vi "AddCustomError.vi"(1 "error in (no error)":errorcluster, 2 "source":string, 3 "code":i32, 4 "Error?":bool) -> (0 "error in (no error) 2":errorcluster)   [LabVIEW 2013]
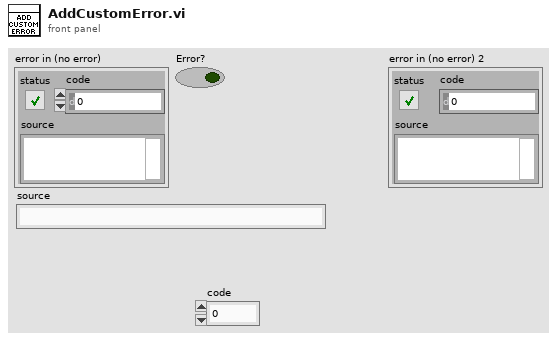
[diagram p1: front panel]
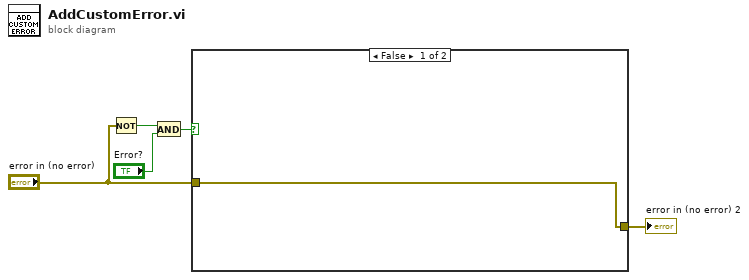
[diagram p0: block diagram]
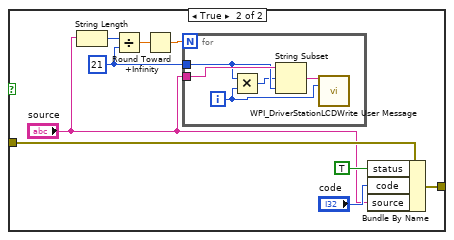
[diagram p2: hidden frame]
diagram:
  n1 = Not(x="error in (no error)") -> (.not. x?=w4:bool)
  n2 = And(x=w4, y="Error?") -> (x .and. y?=w5:bool)
  n3 = case shown="False" w5 {
    tunnel: "error in (no error)" -> [w6 w15]
    tunnel: [w6 w13] -> w1
    frame False {
    }
    frame True {
      w7 = 21 ("y")
      n4 = String Length(string="source") -> (length=w11:i32)
      n5 = Divide(x=w11, y=w7) -> (x/y=w10:dbl)
      n6 = Round Toward +Infinity(x=w10) -> (ceil(x): smallest int >= x=w9:dbl)
      n7 = for {
        N: w9 -> [_]
        tunnel: "source" -> [w20]
        tunnel: w7 -> [w19]
        i -> [w18]
        n8 = Multiply(x=w19, y=w18) -> (x*y=w17:i32)
        n9 = String Subset(string=w20, offset (0)=w17, length (rest)=w19) -> (substring=w16:string)
        n10 = call <vilib>:"WPI_DriverStationLCDWrite User Message.vi"("line text"=w16, "line"=w18) -> ()  [unwired: 13 in, 1 out]
      }
      n11 = Bundle By Name(cluster=w15, "status"=TRUE, "code"="code", "source"="source") -> (w13:errorcluster)
    }
  }
  "error in (no error) 2" <- w1
